vi "Lab2prepare.vi"(0 "String input":string) -> ()   [LabVIEW 2014]
panel:
  out "S":dbl
  out "V":dbl
  out "Hz":dbl
  out "Slope distance":string
  out "Vertical angle":string
  out "Horizontal angle":string
  out "Before sub":string
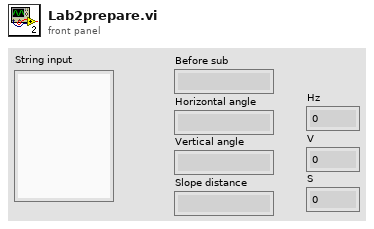
[diagram p1: front panel]
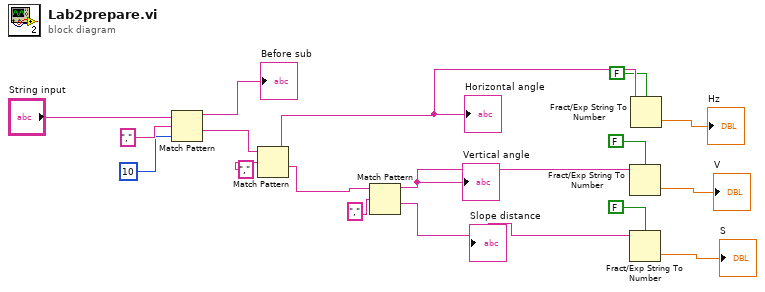
[diagram p0: block diagram]
diagram:
  n1 = Match Pattern(string="String input", regular expression=",", offset (0)=10) -> (before substring=→"Before sub":string, after substring=w12:string)  [unwired: 2 out]
  n2 = Match Pattern(string=w12, regular expression=",") -> (before substring=w9:string, after substring=w10:string)  [unwired: 1 in, 2 out]
  "Horizontal angle" <- w9
  n3 = Match Pattern(string=w10, regular expression=",") -> (before substring=w8:string, after substring=w7:string)  [unwired: 1 in, 2 out]
  "Vertical angle" <- w8
  "Slope distance" <- w7
  n4 = Fract/Exp String To Number(use system decimal point (T)=FALSE, string=w8) -> (number=→"V":dbl)  [unwired: 2 in, 1 out]
  n5 = Fract/Exp String To Number(use system decimal point (T)=FALSE, string=w7) -> (number=→"S":dbl)  [unwired: 2 in, 1 out]
  n6 = Fract/Exp String To Number(use system decimal point (T)=FALSE, string=w9) -> (number=→"Hz":dbl)  [unwired: 2 in, 1 out]
